vi "Error Query.vi"(0 "VISA resource name":refnum<visa-resource-name>, 5 "error in (no error)":errorcluster) -> (14 "VISA resource name out":refnum<visa-resource-name>, 17 "Error":i32, 18 "Error Message":string, 19 "error out":errorcluster)   [LabVIEW 2012, in "Keithley 2000.lvlib"]
doc: "This VI reads an error from the instrument. It expects to see errors in SCPI format (#,\"error message\"). If an error query is not supported, it returns a warning."
uses:
  Keithley 2000.lvlib
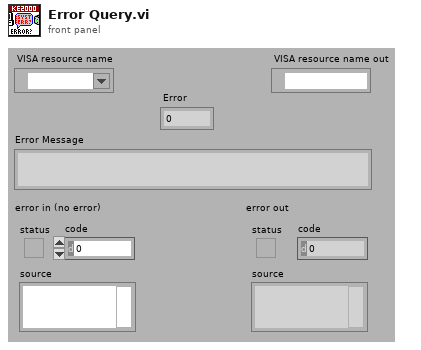
[diagram p1: front panel]
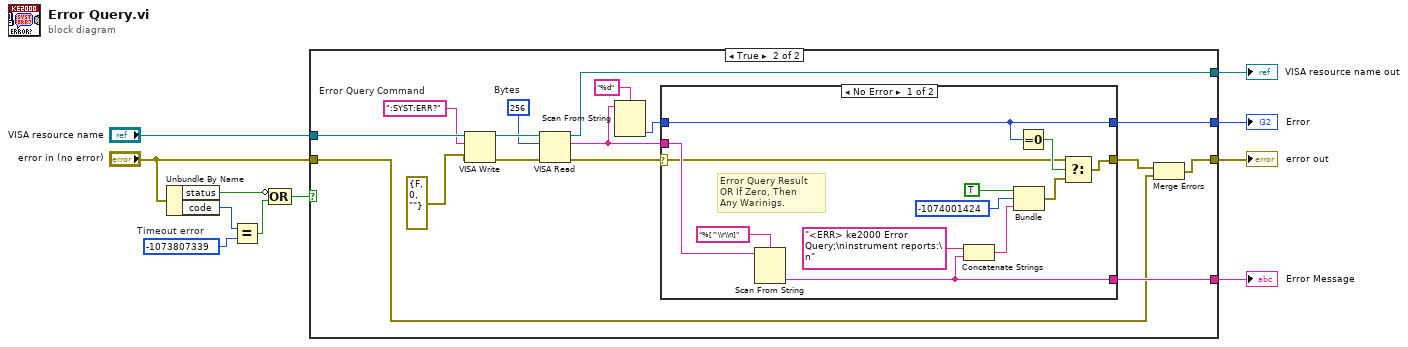
[diagram p0: block diagram]
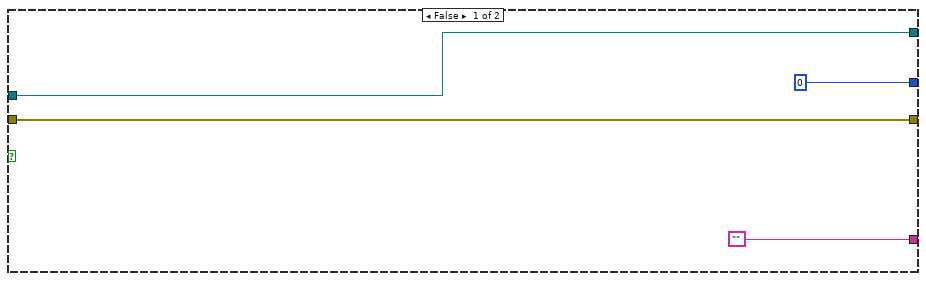
[diagram p2: hidden frame]
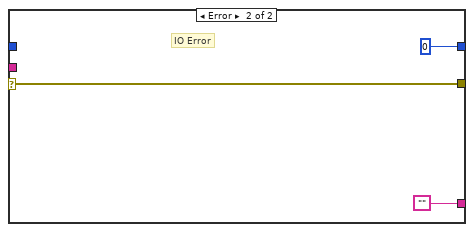
[diagram p3: hidden frame]
diagram:
  w4 = -1073807339  # Timeout error
  n1 = Unbundle By Name("error in (no error)") -> ("status"=w5:bool, "code"=w2:i32)
  n2 = Equal?(x=w2, y=w4) -> (x = y?=w3:bool)
  n3 = Compound Arithmetic op=OR(invert w5, w3) -> (w1:bool)
  n4 = case shown="True" w1 {
    tunnel: ["" w31] -> w11
    tunnel: [0 w30] -> w10
    tunnel: [w15 w29] -> w9
    tunnel: "VISA resource name" -> [w15 w28]
    tunnel: "error in (no error)" -> [w12 w21]
    tunnel: [w12 w20] -> w7
    frame False {
    }
    frame True {
      w26 = u32 256  # Bytes
      w24 = ":SYST:ERR?"  # Error Query Command
      n5 = VISA Write(VISA resource name=w28, write buffer=w24, error in (no error)=errorcluster {"status"=FALSE, "code"=0, "source"=""}) -> (VISA resource name out=w27:refnum<visa-resource-name>, error out=w25:errorcluster)  [unwired: 1 out]
      n6 = VISA Read(VISA resource name=w27, byte count=w26, error in (no error)=w25) -> (VISA resource name out=w29:refnum<visa-resource-name>, read buffer=w19:string, error out=w16:errorcluster)  [unwired: 1 out]
      n7 = Scan From String(format string="%d", input string=w19) -> (output 1=w17:i32)  [unwired: 3 in, 3 out]
      n8 = case shown="No Error" w16 {
        selector: w16 -> [w32 w44]
        tunnel: w19 -> [w34 _]
        tunnel: [w39 w44] -> w22
        tunnel: [w35 ""] -> w31
        tunnel: [w33 0] -> w30
        tunnel: w17 -> [w33 _]
        frame No Error {
          # "Error Query Result\nOR If Zero, Then\nAny Warinigs."
          n9 = Scan From String(format string="%[^\\r\\n]", input string=w34) -> (output 1=w35:string)  [unwired: 3 in, 3 out]
          n10 = Concatenate Strings("<ERR> ke2000 Error Query;\ninstrument reports:\n" ("Source"), w35) -> (w41:string)
          n11 = Bundle("Status"=TRUE, "Code"=-1074001424, w41) -> (w40:cluster{"Status":bool, "Code":i32, string})  [unwired: 1 in]
          n12 = Equal To 0?(x=w33) -> (x = 0?=w37:bool)
          n13 = Select(t=w32, s=w37, f=w40) -> (s? t:f=w39:errorcluster)
        }
        frame Error {
          # "IO Error"
        }
      }
      n14 = Merge Errors(w22, w21) -> (w20:errorcluster)
    }
  }
  "Error Message" <- w11
  "Error" <- w10
  "VISA resource name out" <- w9
  "error out" <- w7
